vi "test_dragon_file--list_vipm_dependencies.vi"(8 "error in (no error)":errorcluster) -> (0 "error out":errorcluster)   [LabVIEW 2020]
uses:
  906ee365-77ae-4f67-adba-29ffbc9f450d.vi
  2bbfc413-0792-4085-b573-6c8503e82316.vi
  baf6d86e-8bd2-4b68-ada5-e98be66b7205.vi
  906ee365-77ae-4f67-adba-29ffbc9f450d.vi/05157253-4ade-4b75-9902-c642c5dd4762.vi
  906ee365-77ae-4f67-adba-29ffbc9f450d.vi/543db544-a529-4041-9332-0fe0cbee0c9f.vi
  2bbfc413-0792-4085-b573-6c8503e82316.vi/05157253-4ade-4b75-9902-c642c5dd4762.vi
  2bbfc413-0792-4085-b573-6c8503e82316.vi/543db544-a529-4041-9332-0fe0cbee0c9f.vi
  baf6d86e-8bd2-4b68-ada5-e98be66b7205.vi/05157253-4ade-4b75-9902-c642c5dd4762.vi
  baf6d86e-8bd2-4b68-ada5-e98be66b7205.vi/543db544-a529-4041-9332-0fe0cbee0c9f.vi
  toml/read_subtable_key_string.vi
  toml/toml.lvclass
  <vilib>/addons/_JKI Toolkits/Caraya/classes/Assert/Assert.lvclass
  <vilib>/addons/_JKI Toolkits/Caraya/classes/Test/Test.lvclass
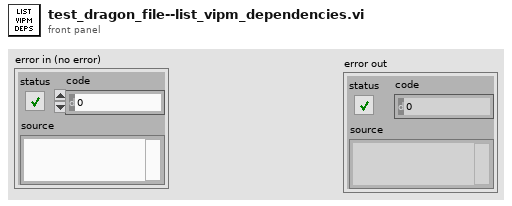
[diagram p1: front panel]
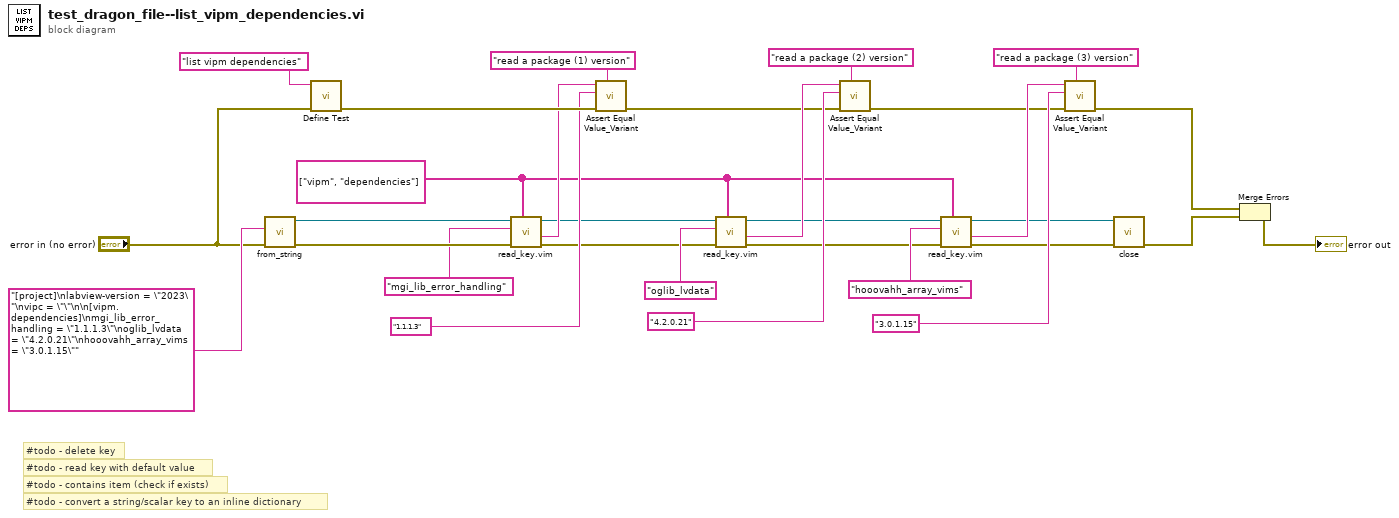
[diagram p0: block diagram]
diagram:
  w6 = string[] ["vipm", "dependencies"]
  # "#todo - contains item (check if exists)"
  # "#todo - convert a string/scalar key to an inline dictionary"
  # "#todo - read key with default value"
  # "#todo - delete key"
  n1 = call "from_string.vi"("error in (no error)"="error in (no error)", "toml"="[project]\nlabview-version = \"2023\"\nvipc = \"\"\n\n[vipm.dependencies]\nmgi_lib_error_handling = \"1.1.1.3\"\noglib_lvdata = \"4.2.0.21\"\nhooovahh_array_vims = \"3.0.1.15\"" ("toml_string in")) -> ("error out"=w24:errorcluster, "toml out"=w25:refnum<class "toml.lvclass">)  [unwired: 8 in]
  n2 = call <vilib>:"Define Test.vi"("error in (no error)"="error in (no error)", "Label (VI Title)"="list vipm dependencies") -> ("error out"=w27:errorcluster)  [unwired: 9 in]
  n3 = call "read_key.vim"("table"=w6, "error in (no error)"=w24, "key"="mgi_lib_error_handling" ("table_name"), "toml in"=w25) -> ("error out"=w12:errorcluster, "value"=w20:string, "toml out"=w13:refnum<class "toml.lvclass">)  [unwired: 4 in, 1 out]
  n4 = call <vilib>:"Assert Equal Value_Variant.vi"("Label"="read a package (1) version", "error in (no error)"=w27, "Y"="1.1.1.3" ("table_name"), "X"=w20) -> ("error out"=w14:errorcluster)  [unwired: 7 in]
  n5 = call "read_key.vim"("table"=w6, "error in (no error)"=w12, "key"="oglib_lvdata" ("table_name"), "toml in"=w13) -> ("error out"=w4:errorcluster, "value"=w17:string, "toml out"=w5:refnum<class "toml.lvclass">)  [unwired: 4 in, 1 out]
  n6 = call <vilib>:"Assert Equal Value_Variant.vi"("Label"="read a package (2) version", "error in (no error)"=w14, "Y"="4.2.0.21" ("table_name"), "X"=w17) -> ("error out"=w7:errorcluster)  [unwired: 7 in]
  n7 = call "read_key.vim"("table"=w6, "error in (no error)"=w4, "key"="hooovahh_array_vims" ("table_name"), "toml in"=w5) -> ("error out"=w2:errorcluster, "value"=w9:string, "toml out"=w3:refnum<class "toml.lvclass">)  [unwired: 4 in, 1 out]
  n8 = call <vilib>:"Assert Equal Value_Variant.vi"("Label"="read a package (3) version", "error in (no error)"=w7, "Y"="3.0.1.15" ("table_name"), "X"=w9) -> ("error out"=w1:errorcluster)  [unwired: 7 in]
  n9 = call "close.vi"("error in (no error)"=w2, "toml in"=w3) -> ("error out"=w23:errorcluster)  [unwired: 9 in]
  n10 = Merge Errors(w1, w23) -> (→"error out":errorcluster)
